vi "BO - Set DIO port A, B, C direction.vi"(1 "Set digital I/O port A and B\ndirection (0 to 3)":string, 3 "error in":errorcluster, 4 "Action":bool, 5 "Address / Port":i16=1 min=1 max=31 step=1) -> (0 "error out":errorcluster, 2 "Report the DIO port\ndirection configuration":string)   [LabVIEW 2014]
panel:
  # "Read"
  # "Write"
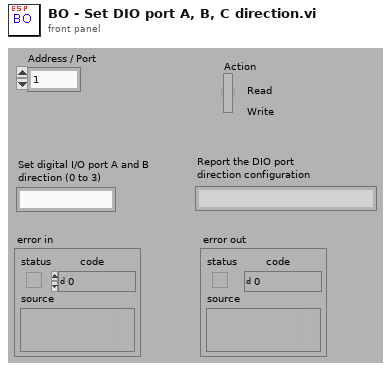
[diagram p1: front panel]
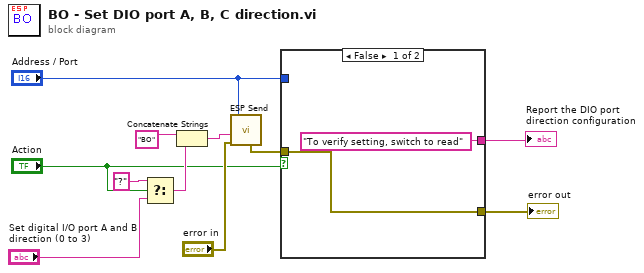
[diagram p0: block diagram]
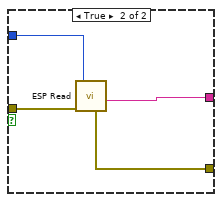
[diagram p2: hidden frame]
diagram:
  n1 = Select(t="?", s="Action", f="Set digital I/O port A and B\ndirection (0 to 3)") -> (s? t:f=w9:string)
  n2 = Concatenate Strings("BO" ("Substring"), w9) -> (w10:string)
  n3 = call "ESP Send.vi"("Address / Port"="Address / Port", "Command String"=w10, "error in"="error in") -> ("error out"=w4:errorcluster)  [unwired: 5 in]
  n4 = case shown="False" "Action" {
    tunnel: "Address / Port" -> [_ w17]
    tunnel: w4 -> [w13 w16]
    tunnel: [w13 w15] -> w3
    tunnel: ["To verify setting, switch to read" w14] -> w2
    frame False {
    }
    frame True {
      n5 = call "ESP Read.vi"("Address / Port"=w17, "error in"=w16) -> ("error out"=w15:errorcluster, "Response String"=w14:string)  [unwired: 5 in]
    }
  }
  "error out" <- w3
  "Report the DIO port\ndirection configuration" <- w2
